vi "write.vi"(8 "错误输入（无错误）":errorcluster, 10 "Write Buffer":string="SENS:DATA?" caption="写入缓冲区", 11 "VISA GPIB Resource":refnum<visa-resource-name>="GPIB0::2::INSTR" caption="VISA GPIB资源") -> (0 "错误输出":errorcluster, 3 "VISA资源名称输出":refnum<visa-resource-name>)   [LabVIEW 2017]
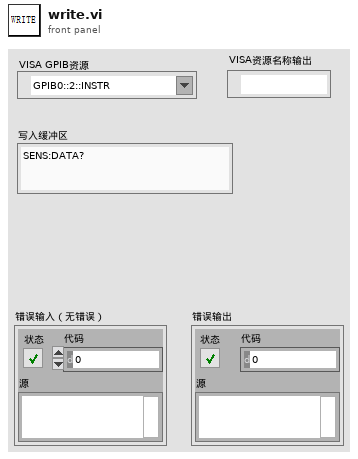
[diagram p1: front panel]
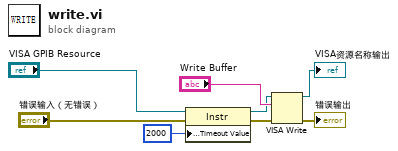
[diagram p0: block diagram]
diagram:
  n1 = property class="Instr"(reference="VISA GPIB Resource", error in="错误输入（无错误）", "General Settings:Timeout Value"=u32 2000) -> (reference out=w6:refnum<visa-resource-name>, error out=w5:errorcluster)
  n2 = VISA Write(VISA resource name=w6, write buffer="Write Buffer", error in (no error)=w5) -> (VISA resource name out=→"VISA资源名称输出":refnum<visa-resource-name>, error out=→"错误输出":errorcluster)  [unwired: 1 out]
